vi "数据查询_数据查询.vi"() -> ()   [LabVIEW 2016]
uses:
  <vilib>/Utility/miscctls.llb/LVPointTypeDef.ctl
  <vilib>/Utility/miscctls.llb/LVRowAndColumnUnsignedTypeDef.ctl
  <userlib>/_OpenG.lib/array/array.llb/Sort 2D Array (String)__ogtk.vi
  <vilib>/addons/database/_DB Variant To Data/Database Variant To Data.xnode
panel:
  in  "是否剔除异常数据":bool=TRUE
  in  "下拉列表":string(xcontrol)
  in  "导出":bool
  out "分钟小时":string(combo)="实时数据"
  out "工作类型":string(combo)="全部数据"
  out "连接的字符串":string
  out "选中数据表":string
  in  "查询":bool
  in  "结束日期":string="2050/01/01"
  in  "起始日期":string="2010/01/01"
  out "XY图":cluster{"data":timestamp[], "data":dbl[]}[](graph)
  out "数据表":string[][](table)
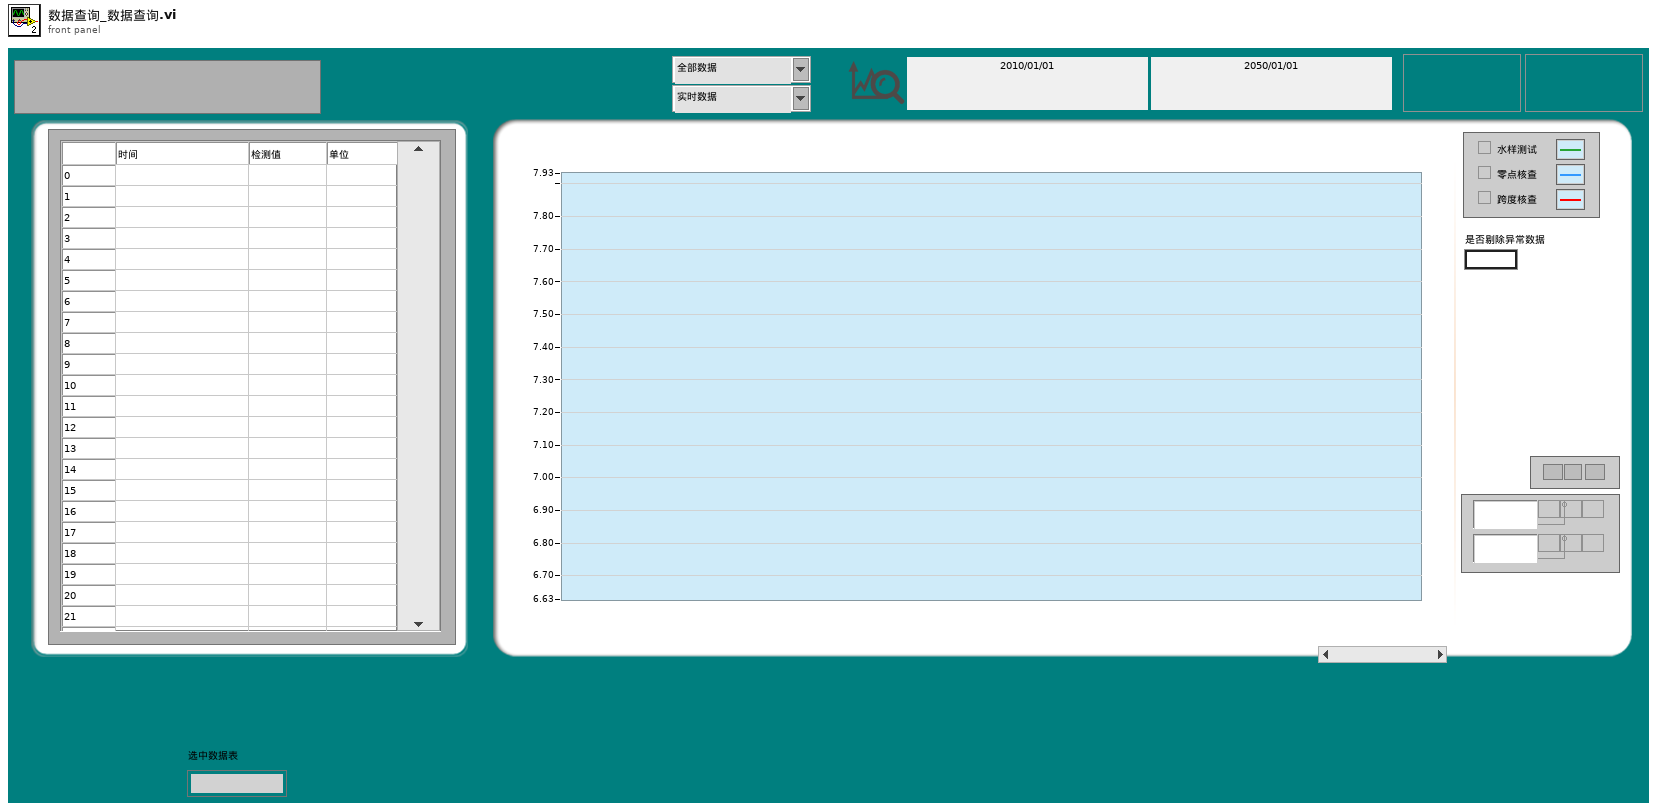
[diagram p1: front panel]
types:
  T1 = typedef "LVPointTypeDef.ctl" = cluster{"Horizontal":i16, "Vertical":i16}
  T2 = typedef "LVDateTimeRec.ctl" = cluster{"秒数的小数部分":dbl, "秒":i32, "分":i32, "时":i32, "日":i32, "月":i32, "年":i32, "天数（周）":i32, "天数（年）":i32, "DST":i32}
  T3 = enum8{"Enabled", "Disabled", "Disabled and Grayed Out"}
  T4 = typedef "LVPoint32TypeDef.ctl" = cluster{"Horizontal":i32, "Vertical":i32}
  T5 = typedef "LVPointDoubleTypeDef.ctl" = cluster{"Cursor X":dbl, "Cursor Y":dbl}
  T6 = typedef "LVRowAndColumnUnsignedTypeDef.ctl" = cluster{"Row":u32, "Column":u32}
  T7 = cluster{"时间":timestamp, "检测值":dbl, "单位":string, "测量模式":string}[]
  T8 = cluster{"时间":timestamp, "检测值":dbl, "单位":string}[]
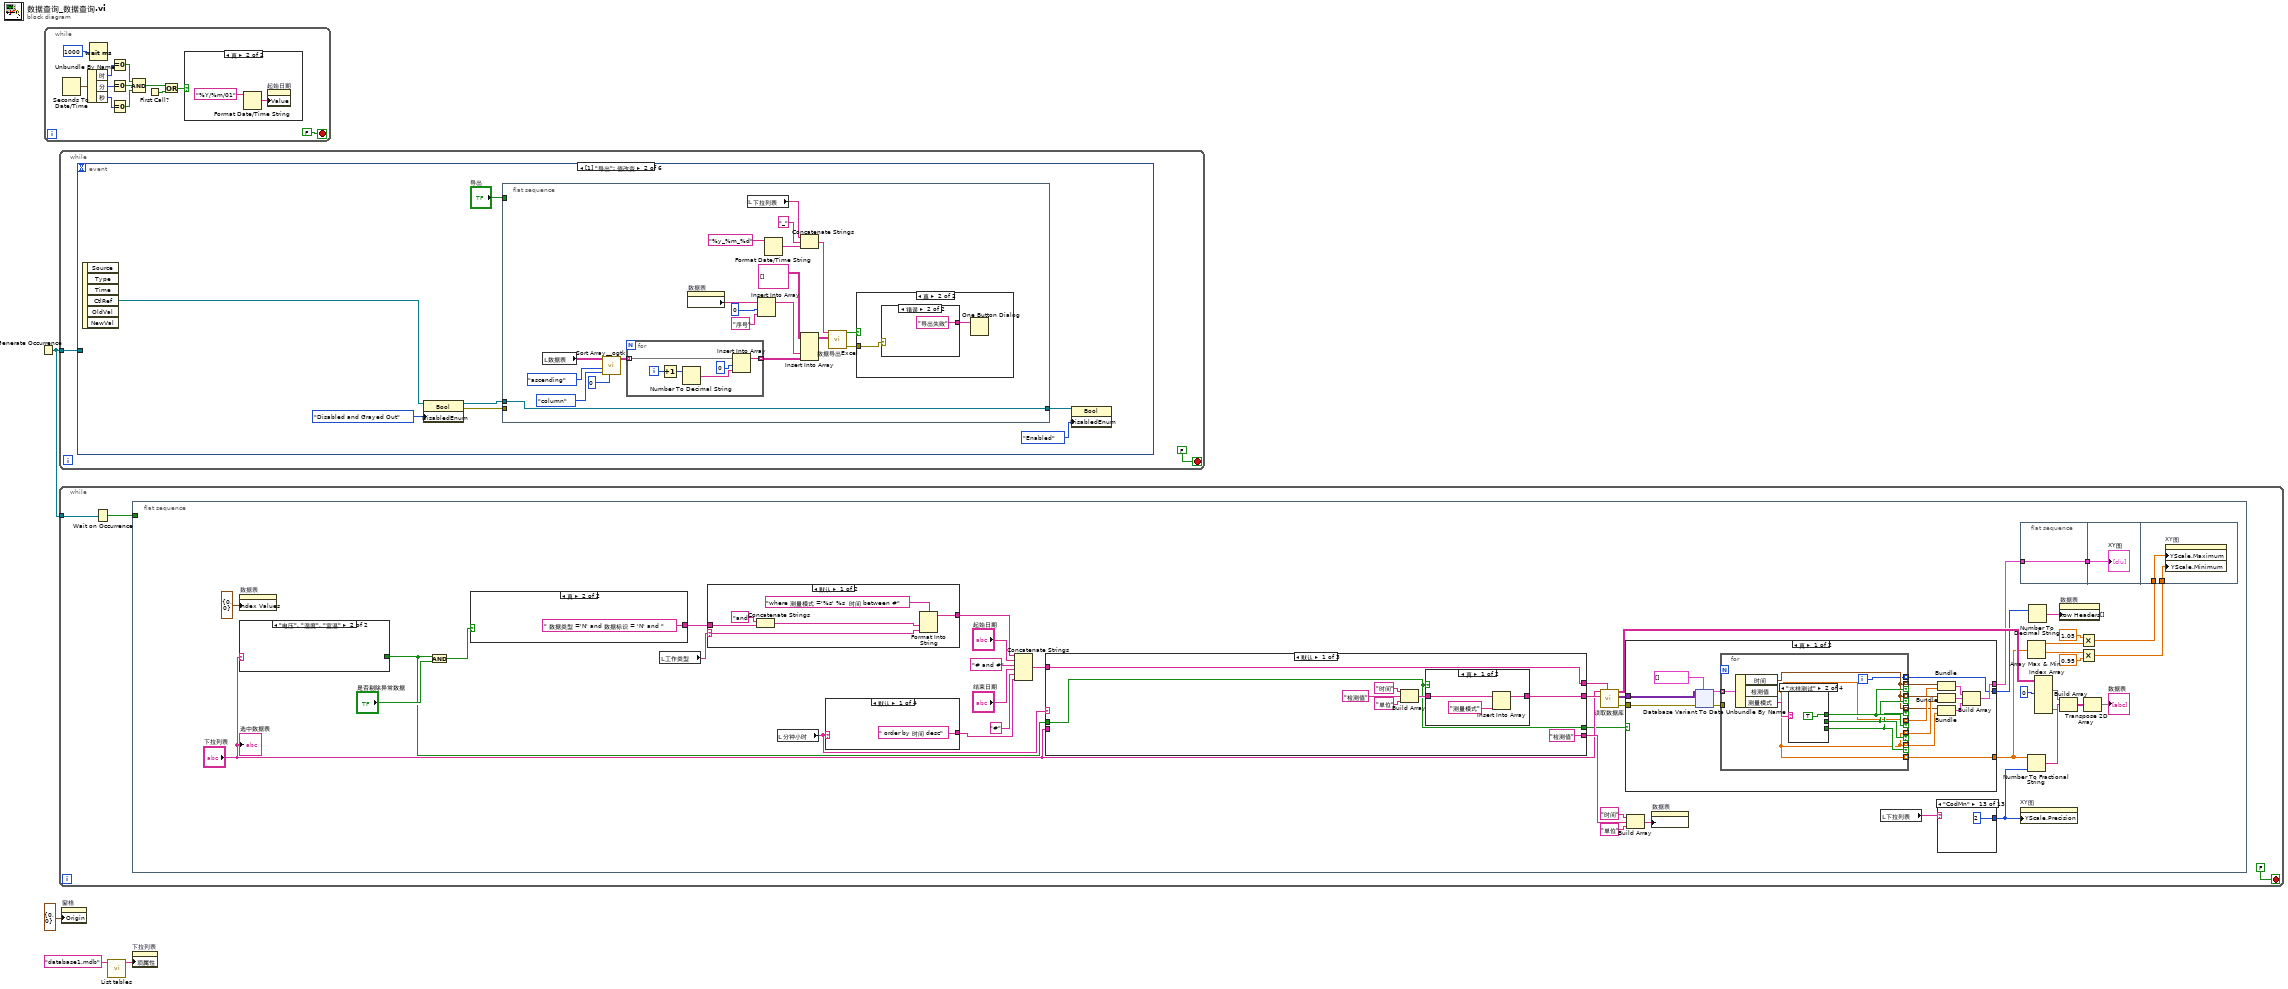
[diagram p0: block diagram]
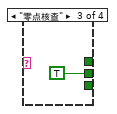
[diagram p3: hidden frame]
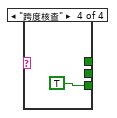
[diagram p4: hidden frame]
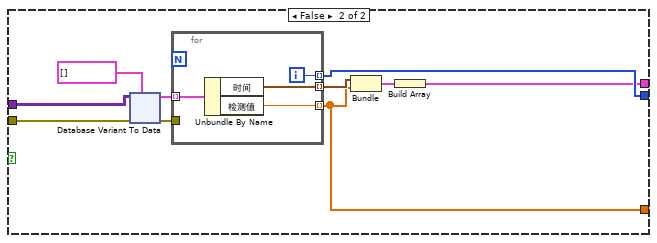
[diagram p5: hidden frame]
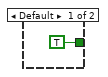
[diagram p6: hidden frame]
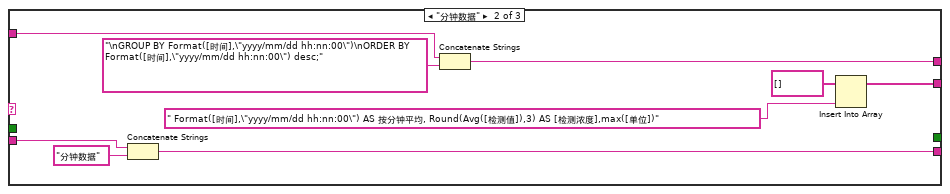
[diagram p9: hidden frame]
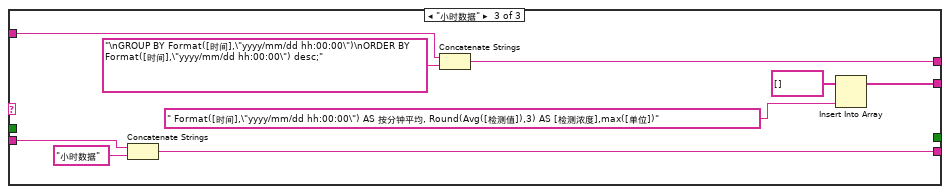
[diagram p10: hidden frame]
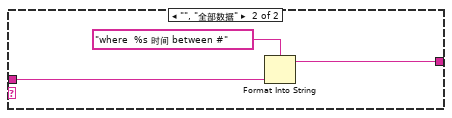
[diagram p14: hidden frame]
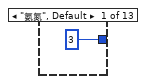
[diagram p15: hidden frame]
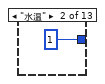
[diagram p16: hidden frame]
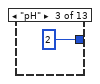
[diagram p17: hidden frame]
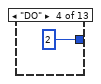
[diagram p18: hidden frame]
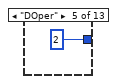
[diagram p19: hidden frame]
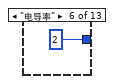
[diagram p20: hidden frame]
diagram:
  n1 = Generate Occurrence() -> (w1:refnum<k4>)
  n2 = while {
    stop <- FALSE stop-if-true
    n3 = Seconds To Date/Time() -> (date time rec=w16:T2)  [unwired: 2 in]
    n4 = Unbundle By Name(w16) -> ("时"=w15:i32, "分"=w14:i32, "秒"=w13:i32)
    n5 = Wait (ms)(milliseconds to wait=u32 1000 ("等待时间（毫秒）")) -> ()  [unwired: 1 out]
    n6 = Equal To 0?(x=w15) -> (x = 0?=w12:bool)
    n7 = Equal To 0?(x=w14) -> (x = 0?=w11:bool)
    n8 = Equal To 0?(x=w13) -> (x = 0?=w10:bool)
    n9 = Compound Arithmetic op=AND ("复合运算")(w12, w11, w10) -> (w7:bool)
    n10 = First Call?() -> (First Call?: T/F=w5:bool)
    n11 = Or(x=w7, y=w5) -> (x .or. y?=w6:bool)
    n12 = case shown="真" w6 {
      frame False {
      }
      frame True {
        n13 = Format Date/Time String(time format string (%c)="%Y/%m/01" ("时间格式字符串(%c)")) -> (date/time string=w17:string)  [unwired: 2 in]
        n14 = property on="起始日期" class="Str"("Value"=w17) -> ()  [unwired: 2 in, 2 out]
      }
    }
  }
  n15 = while {
    tunnel: w1 -> [w19]
    stop <- FALSE stop-if-true
    n16 = event shown="[1] \"导出\": 值改变" {
      selector: _ -> [_ _ _ _ _ _]
      dyn-events: _ -> [_ _ _ _ _ _]
      timeout: _ -> [_ _ _ _ _ _]
      tunnel: w19 -> [_ _ _ _ w64 _]
      event Timeout {
        n17 = event-data() -> ()  [unwired: 1 in, 3 out]
      }
      event "导出": Value Change {
        n18 = event-data() -> ("CtlRef"=w27:refnum<vi>)  [unwired: 1 in, 5 out]
        n19 = property class="Bool"(reference=w27, "DisabledEnum"=T3."Disabled and Grayed Out" ("禁用")) -> (reference out=w24:refnum<vi>, error out=w25:errorcluster)  [unwired: 1 in]
        n20 = flat-sequence {
          tunnel: w25 -> [_]
          tunnel: [w43] -> w23
          tunnel: w24 -> [w43]
          tunnel: "导出" -> [_]
          frame #0 {
            n21 = local read "数据表"() -> (w47:string[][])
            n22 = call-poly <userlib>:"Sort Array__ogtk.vi"("Column/Row to Sort By"=u32 0, "Sort By in"=enum16{"row", "column"}."column", "Order"=enum16{"ascending", "descending"}."ascending", "Array in"=w47) -> ("Sorted Array out"=w36:string[][])  [unwired: 4 in, 3 out]
            n23 = for {
              tunnel: w36 -> [w56] mode=indexing
              tunnel: [w55] -> w31 mode=indexing
              i -> [w57]
              n24 = Increment(x=w57) -> (x+1=w53:i32)
              n25 = Number To Decimal String(number=w53) -> (decimal integer string=w52:string)  [unwired: 1 in]
              n26 = Insert Into Array(array=w56, index=0 ("索引"), new element=w52) -> (w55:string[])
            }
            n27 = property on="数据表" class="Tbl (严格)"() -> ("Column Headers[]"=w34:string[])  [unwired: 2 in, 2 out]
            n28 = local read "下拉列表"() -> (w39:string)
            n29 = Insert Into Array(array=w34, index=0 ("索引"), new element="序号" ("新元素/子数组")) -> (w35:string[])
            n30 = Format Date/Time String(time format string (%c)="%y_%m_%d" ("时间格式字符串(%c)")) -> (date/time string=w40:string)  [unwired: 2 in]
            n31 = Concatenate Strings(w39, "_" ("字符串"), w40) -> (w37:string)
            n32 = Insert Into Array(array=string[][] [], new element #1=w35, new element #2=w31) -> (w30:string[][])  [unwired: 2 in]
            n33 = call "数据导出Excel.vi"("text data"=w30, "default name"=w37) -> ("error out"=w29:errorcluster, "布尔"=w28:bool)  [unwired: 8 in]
            n34 = case shown="真" w28 {
              tunnel: w29 -> [_ w49]
              frame False {
              }
              frame True {
                n35 = case shown="错误" w49 {
                  tunnel: ["导出成功" ("消息") "导出失败" ("消息")] -> w48
                  frame No Error {
                  }
                  frame Error {
                  }
                }
                n36 = One Button Dialog(message=w48) -> ()  [unwired: 1 in, 1 out]
              }
            }
          }
        }
        n37 = property class="Bool"(reference=w23, "DisabledEnum"=T3."Enabled" ("禁用")) -> ()  [unwired: 1 in, 2 out]
      }
      event "工作类型", "分钟小时": Mouse Down {
        n38 = event-data() -> ()  [unwired: 1 in, 8 out]
        n39 = call "数据查询筛选.vi"() -> ("分钟小时"=→"分钟小时":string, "工作类型"=w58:string)  [unwired: 10 in]
        n40 = property on="工作类型" class="CmbBox"("Val(Sgnl)"=w58) -> ()  [unwired: 2 in, 2 out]
      }
      event "起始日期", "结束日期": Mouse Down {
        n41 = event-data() -> ("CtlRef"=w63:refnum<vi>)  [unwired: 1 in, 7 out]
        n42 = property class="Str"(reference=w63) -> (reference out=w61:refnum<vi>, "Value"=w62:string)  [unwired: 1 in, 1 out]
        n43 = call "日期键盘.vi"("原值"=w62) -> ("x+y"=w60:string)  [unwired: 10 in]
        n44 = property class="Str"(reference=w61, "Val(Sgnl)"=w60) -> ()  [unwired: 1 in, 2 out]
      }
      event "查询", "下拉列表", "起始日期", "结束日期", "工作类型", "分钟小时": Value Change {
        n45 = event-data() -> ()  [unwired: 1 in, 6 out]
        n46 = Set Occurrence(w64) -> ()
        n47 = call "List tables.vi"("database"="database1.mdb") -> ("tables"=w65:string[])  [unwired: 9 in, 1 out]
        n48 = property on="下拉列表" class="下拉列表 (严格)"("项属性"=w65) -> ()  [unwired: 2 in, 2 out]
      }
      event "XY图": Mouse Move {
        w70 = "   " ("字符串")
        n49 = event-data() -> ("CtlRef"=w80:refnum<vi>, "Coords"=w79:T4)  [unwired: 1 in, 3 out]
        n50 = invoke class="XYGraph (严格)" method="Map Coords To XY"(reference=w80, "Coords"=w79) -> (reference out=w78:refnum<vi>, error out=w75:errorcluster, "XY"=w77:cluster{"X":dbl, "Y":dbl})  [unwired: 5 in, 4 out]
        n51 = property class="XYGraph (严格)"(reference=w78, error in=w75, "Cursor.Cursor Position"=w77) -> (error out=w76:errorcluster)  [unwired: 1 out]
        n52 = property on="XY图" class="XYGraph (严格)" props=["Cursor", "Cursor Position", "YScale", "Precision", "CrsrList"](error in=w76) -> ("Cursor.Cursor Position"=w73:T5, "YScale.Precision"=w67:u8)  [unwired: 1 in, 3 out]
        n53 = Unbundle(w73) -> ("Cursor X"=w72:dbl, "Cursor Y"=w69:dbl)
        n54 = Number To Fractional String(number=w69, precision (6)=w67) -> (F-format string=w68:string)  [unwired: 2 in]
        n55 = Format Date/Time String(seconds (now)=w72) -> (date/time string=w71:string)  [unwired: 2 in]
        n56 = Concatenate Strings(w70, w71, w70, w68) -> (→"连接的字符串":string)
      }
    }
  }
  n57 = while {
    tunnel: w1 -> [w82]
    stop <- FALSE stop-if-true
    n58 = Wait on Occurrence(2:w82) -> (0:w81:bool)  [unwired: 2 in]
    n59 = flat-sequence {
      tunnel: w81 -> [_]
      frame #0 {
        n60 = property on="数据表" class="Tbl (严格)"("Index Values"=T6 {"Row"=0, "Column"=0} ("索引值")) -> ()  [unwired: 2 in, 2 out]
        n61 = case shown="\"电压\", \"湿度\", \"室温\"" "下拉列表" {
          tunnel: [TRUE _] -> w86
          frame Default {
          }
          frame "电压", "湿度", "室温" {
          }
        }
        n62 = And(x=w86, y="是否剔除异常数据") -> (x .and. y?=w87:bool)
        n63 = case shown="真" w87 {
          tunnel: [_ " 数据类型 ='N' and 数据标识 = 'N' and " ("condition")] -> w97
          frame False {
          }
          frame True {
          }
        }
        n64 = local read "工作类型"() -> (w118:string)
        n65 = case shown="默认" w118 {
          selector: w118 -> [w471 _]
          tunnel: [w469 w473] -> w119
          tunnel: w97 -> [w468 w472]
          frame Default {
            n66 = Concatenate Strings("and" ("字符串"), w468) -> (w467:string)
            n67 = Format Into String(format string="where 测量模式 ='%s' %s  时间 between #" ("condition"), w467, w471) -> (resulting string=w469:string)  [unwired: 2 in, 1 out]
          }
          frame "", "全部数据" {
            n68 = Format Into String(format string="where  %s 时间 between #" ("condition"), w472) -> (resulting string=w473:string)  [unwired: 2 in, 1 out]
          }
        }
        n69 = local read "分钟小时"() -> (w122:string)
        n70 = case shown="默认" w122 {
          tunnel: [" order by 时间 desc" ("字符串") _ _ _] -> w120
          frame Default {
          }
          frame "分钟数据" {
          }
          frame "小时数据" {
          }
          frame "真" {
          }
        }
        n71 = Concatenate Strings(w119, "起始日期", "# and #" ("condition"), "结束日期", "#" ("condition"), w120) -> (w121:string)
        n72 = case shown="默认" w122 {
          tunnel: [w436 w454 w459] -> w124
          tunnel: w121 -> [w442 w452 w461]
          tunnel: [w442 w451 w460] -> w123
          tunnel: ["检测值" w447 w456] -> w125
          tunnel: "下拉列表" -> [_ w448 w458]
          tunnel: w86 -> [w435 _ _]
          tunnel: [w435 _ _] -> w84
          frame Default {
            n73 = Build Array("时间", "检测值", "单位" ("元素")) -> (w437:string[])
            n74 = case shown="真" w435 {
              tunnel: w437 -> [w445 w446]
              tunnel: [w443 w446] -> w436
              frame True {
                n75 = Insert Into Array(array=w445, new element="测量模式" ("元素")) -> (w443:string[])  [unwired: 1 in]
              }
              frame False {
              }
            }
          }
          frame "分钟数据" {
            n76 = Concatenate Strings(w448, "分钟数据" ("字符串")) -> (w447:string)
            n77 = Concatenate Strings(w452, "\nGROUP BY Format([时间],\"yyyy/mm/dd hh:nn:00\")\nORDER BY Format([时间],\"yyyy/mm/dd hh:nn:00\") desc;" ("字符串")) -> (w451:string)
            n78 = Insert Into Array(array=string[] [] ("显示项"), new element=" Format([时间],\"yyyy/mm/dd hh:nn:00\") AS 按分钟平均, Round(Avg([检测值]),3) AS [检测浓度],max([单位])" ("新元素/子数组")) -> (w454:string[])  [unwired: 1 in]
          }
          frame "小时数据" {
            n79 = Concatenate Strings(w458, "小时数据" ("字符串")) -> (w456:string)
            n80 = Concatenate Strings(w461, "\nGROUP BY Format([时间],\"yyyy/mm/dd hh:00:00\")\nORDER BY Format([时间],\"yyyy/mm/dd hh:00:00\") desc;" ("字符串")) -> (w460:string)
            n81 = Insert Into Array(array=string[] [] ("显示项"), new element=" Format([时间],\"yyyy/mm/dd hh:00:00\") AS 按分钟平均, Round(Avg([检测值]),3) AS [检测浓度],max([单位])" ("新元素/子数组")) -> (w459:string[])  [unwired: 1 in]
          }
        }
        n82 = call "读取数据库.vi"("condition"=w123, "显示项"=w124, "组合框"="下拉列表") -> ("error out"=w96:errorcluster, "data"=w85:variant[][], "表格"=w104:string[][])  [unwired: 5 in, 1 out]
        n83 = case shown="真" w84 {
          tunnel: w96 -> [w144 w312]
          tunnel: [w131 w303] -> w95
          tunnel: [w130 w307] -> w94
          tunnel: [w129 w305] -> w93
          tunnel: w85 -> [w128 w306]
          frame True {
            n84 = xnode "Database Variant To Data"("database variant"=w128, "error in (no error)"=w144, "type"=T7 []) -> ("data"=w141:T7, "error out"=w142:errorcluster)
            n85 = for {
              tunnel: w141 -> [w152] mode=indexing
              tunnel: w142 -> [_]
              tunnel: [w148] -> w137 mode=indexing if=w150
              tunnel: [w146] -> w138 mode=indexing if=w150
              tunnel: [w148] -> w140 mode=indexing if=w149
              tunnel: [w146] -> w139 mode=indexing if=w149
              tunnel: [w148] -> w136 mode=indexing if=w147
              tunnel: [w146] -> w135 mode=indexing if=w147
              tunnel: [w146] -> w129 mode=indexing
              tunnel: [w145] -> w130 mode=indexing
              i -> [w145]
              n86 = Unbundle By Name(w152) -> ("时间"=w148:timestamp, "检测值"=w146:dbl, "测量模式"=w151:string)
              n87 = case shown="\"水样测试\"" w151 {
                tunnel: [_ TRUE _ _] -> w150
                tunnel: [_ _ TRUE _] -> w149
                tunnel: [_ _ _ TRUE] -> w147
                frame "假", Default {
                }
                frame "水样测试" {
                }
                frame "零点核查" {
                }
                frame "跨度核查" {
                }
              }
            }
            n88 = Bundle(w137, w138) -> (w134:cluster{timestamp[], dbl[]})  [unwired: 1 in]
            n89 = Bundle(w140, w139) -> (w133:cluster{timestamp[], dbl[]})  [unwired: 1 in]
            n90 = Bundle(w136, w135) -> (w132:cluster{timestamp[], dbl[]})  [unwired: 1 in]
            n91 = Build Array(w134, w133, w132) -> (w131:cluster{timestamp[], dbl[]}[])
          }
          frame False {
            n92 = xnode "Database Variant To Data"("database variant"=w306, "error in (no error)"=w312, "type"=T8 []) -> ("data"=w309:T8, "error out"=w310:errorcluster)
            n93 = for {
              tunnel: w309 -> [w316] mode=indexing
              tunnel: w310 -> [_]
              tunnel: [w315] -> w308 mode=indexing
              tunnel: [w314] -> w305 mode=indexing
              tunnel: [w313] -> w307 mode=indexing
              i -> [w313]
              n94 = Unbundle By Name(w316) -> ("时间"=w315:timestamp, "检测值"=w314:dbl)
            }
            n95 = Bundle(w308, w305) -> (w304:cluster{timestamp[], dbl[]})  [unwired: 1 in]
            n96 = Build Array(w304) -> (w303:cluster{timestamp[], dbl[]}[])
          }
        }
        n97 = Build Array("时间", w125, "单位" ("元素")) -> (w110:string[])
        n98 = property on="数据表" class="Tbl (严格)"("Column Headers[]"=w110) -> ()  [unwired: 2 in, 2 out]
        n99 = local read "下拉列表"() -> (w114:string)
        n100 = case shown="\"CodMn\"" w114 {
          tunnel: [i16 3 ("精度(6)") i16 1 ("精度(6)") i16 2 ("精度(6)") i16 2 ("精度(6)") i16 2 ("精度(6)") i16 2 ("精度(6)") i16 2 ("精度(6)") i16 2 ("精度(6)") i16 2 ("精度(6)") i16 3 ("精度(6)") i16 2 ("精度(6)") i16 2 ("精度(6)") i16 2 ("精度(6)")] -> w117
          frame "氨氮", Default {
          }
          frame "水温" {
          }
          frame "pH" {
          }
          frame "DO" {
          }
          frame "DOper" {
          }
          frame "电导率" {
          }
          frame "浊度" {
          }
          frame "藻密度" {
          }
          frame "叶绿素a" {
          }
          frame "总磷" {
          }
          frame "总氮" {
          }
          frame "CodCr" {
          }
          frame "CodMn" {
          }
        }
        n101 = flat-sequence {
          tunnel: [w488] -> w127
          tunnel: w95 -> [w488]
          tunnel: w127 -> [w489]
          tunnel: w92 -> [w491]
          tunnel: w90 -> [w490]
          frame #0 {
          }
          frame #1 {
            "XY图" <- w489
          }
          frame #2 {
            n102 = property on="XY图" class="XYGraph (严格)"("YScale.Maximum"=w491, "YScale.Minimum"=w490) -> ()  [unwired: 2 in, 2 out]
          }
        }
        n103 = property on="XY图" class="XYGraph (严格)"("YScale.Precision"=w117) -> ()  [unwired: 2 in, 2 out]
        n104 = Array Max & Min(array=w93) -> (max value=w115:dbl, min value=w116:dbl)  [unwired: 2 out]
        n105 = Number To Fractional String(number=w93, precision (6)=w117) -> (F-format string=w113:string[])  [unwired: 2 in]
        n106 = Number To Decimal String(number=w94) -> (decimal integer string=w126:string[])  [unwired: 1 in]
        n107 = Index Array(array=w104, index (col) #1=0 ("禁用的索引 (列)")) -> (element #1=w106:string[], element #3=w112:string[])  [unwired: 5 in, 1 out]
        n108 = property on="数据表" class="Tbl (严格)"("Row Headers[]"=w126) -> ()  [unwired: 2 in, 2 out]
        n109 = Build Array(w106, w113, w112) -> (w107:string[][])
        n110 = Multiply(x=1.05, y=w115) -> (x*y=w92:dbl)
        n111 = Multiply(x=w116, y=0.95) -> (x*y=w90:dbl)
        n112 = Transpose 2D Array(2D array=w107) -> (transposed array=→"数据表":string[][])
        "选中数据表" <- "下拉列表"
      }
    }
  }
  n113 = property on="窗格" class="Pane"("Origin"=T1 {"Horizontal"=0, "Vertical"=0} ("原点")) -> ()  [unwired: 2 in, 2 out]
  n114 = call "List tables.vi"("database"="database1.mdb") -> ("tables"=w2:string[])  [unwired: 9 in, 1 out]
  n115 = property on="下拉列表" class="下拉列表 (严格)"("项属性"=w2) -> ()  [unwired: 2 in, 2 out]
